vi "Send to Logger.vi"(6 "dt":dbl, 8 "error in (no error)":errorcluster, 9 "t0":dbl, 10 "Data":dbl[][](array[numeric]), 11 "DataProcessor in":refnum<class "DataProcessor.lvclass">) -> (0 "error out":errorcluster, 3 "DataProcessor out":refnum<class "DataProcessor.lvclass">)   [LabVIEW 2020, in "VolatusData.lvlib" / "DataProcessor.lvclass"]
uses:
  DataProcessor.lvclass
  DataProcessor.lvclass/DataProcessor.ctl
  DataHandlerAPI/DataHandlerAPI.lvclass/DataHandlerAPI.ctl
  DataHandler Messages/New Data Msg/New Data Msg.lvclass/New Data Msg.ctl
  <vilib>/ActorFramework/Message Enqueuer/Message Enqueuer.lvclass/Message Enqueuer.ctl
  DataHandler Messages/New Data Msg/Send New Data.vi
  <vilib>/ActorFramework/Message Enqueuer/Enqueue.vi
  DataHandler Messages/New Data Msg/New Data Msg.lvclass
  C:/Program Files (x86)/National Instruments/LabVIEW 2020/vi.lib/ActorFramework/Message/Message.lvclass
  <vilib>/ActorFramework/Message Priority Queue/Priority Enqueue.vi
  DataHandlerAPI/DataHandlerAPI.lvclass
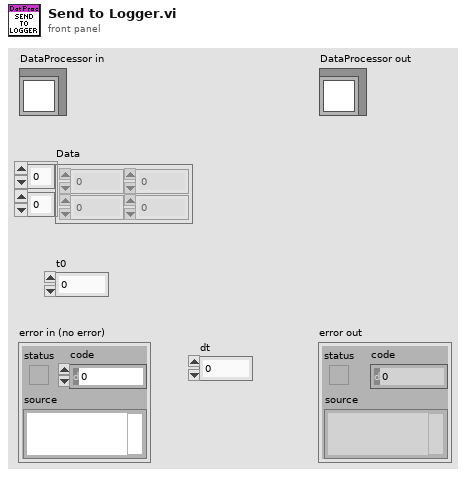
[diagram p1: front panel]
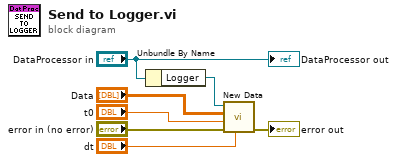
[diagram p0: block diagram]
diagram:
  n1 = Unbundle By Name("DataProcessor in") -> ("Logger"=w2:refnum<class "DataHandlerAPI.lvclass">)
  n2 = call "New Data.vi"("dt"="dt", "error in (no error)"="error in (no error)", "t0"="t0", "Data"="Data", "DataHandlerAPI in"=w2) -> ("error out"=→"error out":errorcluster)  [unwired: 5 in, 1 out]
  "DataProcessor out" <- "DataProcessor in"
